vi "Buffer.vi"(7 "Cluster":T1={"JSON Buffer"="authtoken=239cf72879e39d0ce6e668cd5c3988b6&scope=creatorapi&zc_ownername=shanthapriya&XMLString=", "Server information start tag"="<ZohoCreator> <applicationlist> <application name='customer-application'><formlist>  <form name='EventLog'>", "Record start/end"="add", "Key name"="field name", "Value name"="value", "Server information end tag"="\"</form></formlist></application></applicationlist></ZohoCreator>"}, 8 "error in":errorcluster, 10 "Values":string[][](array[string]), 11 "Keys":string[](array[string])) -> (0 "Error out":errorcluster, 3 "Buffer":string)   [LabVIEW 2019, in "DataLogger.lvclass"]
doc: "Buffer"
uses:
  DataLogger.lvclass
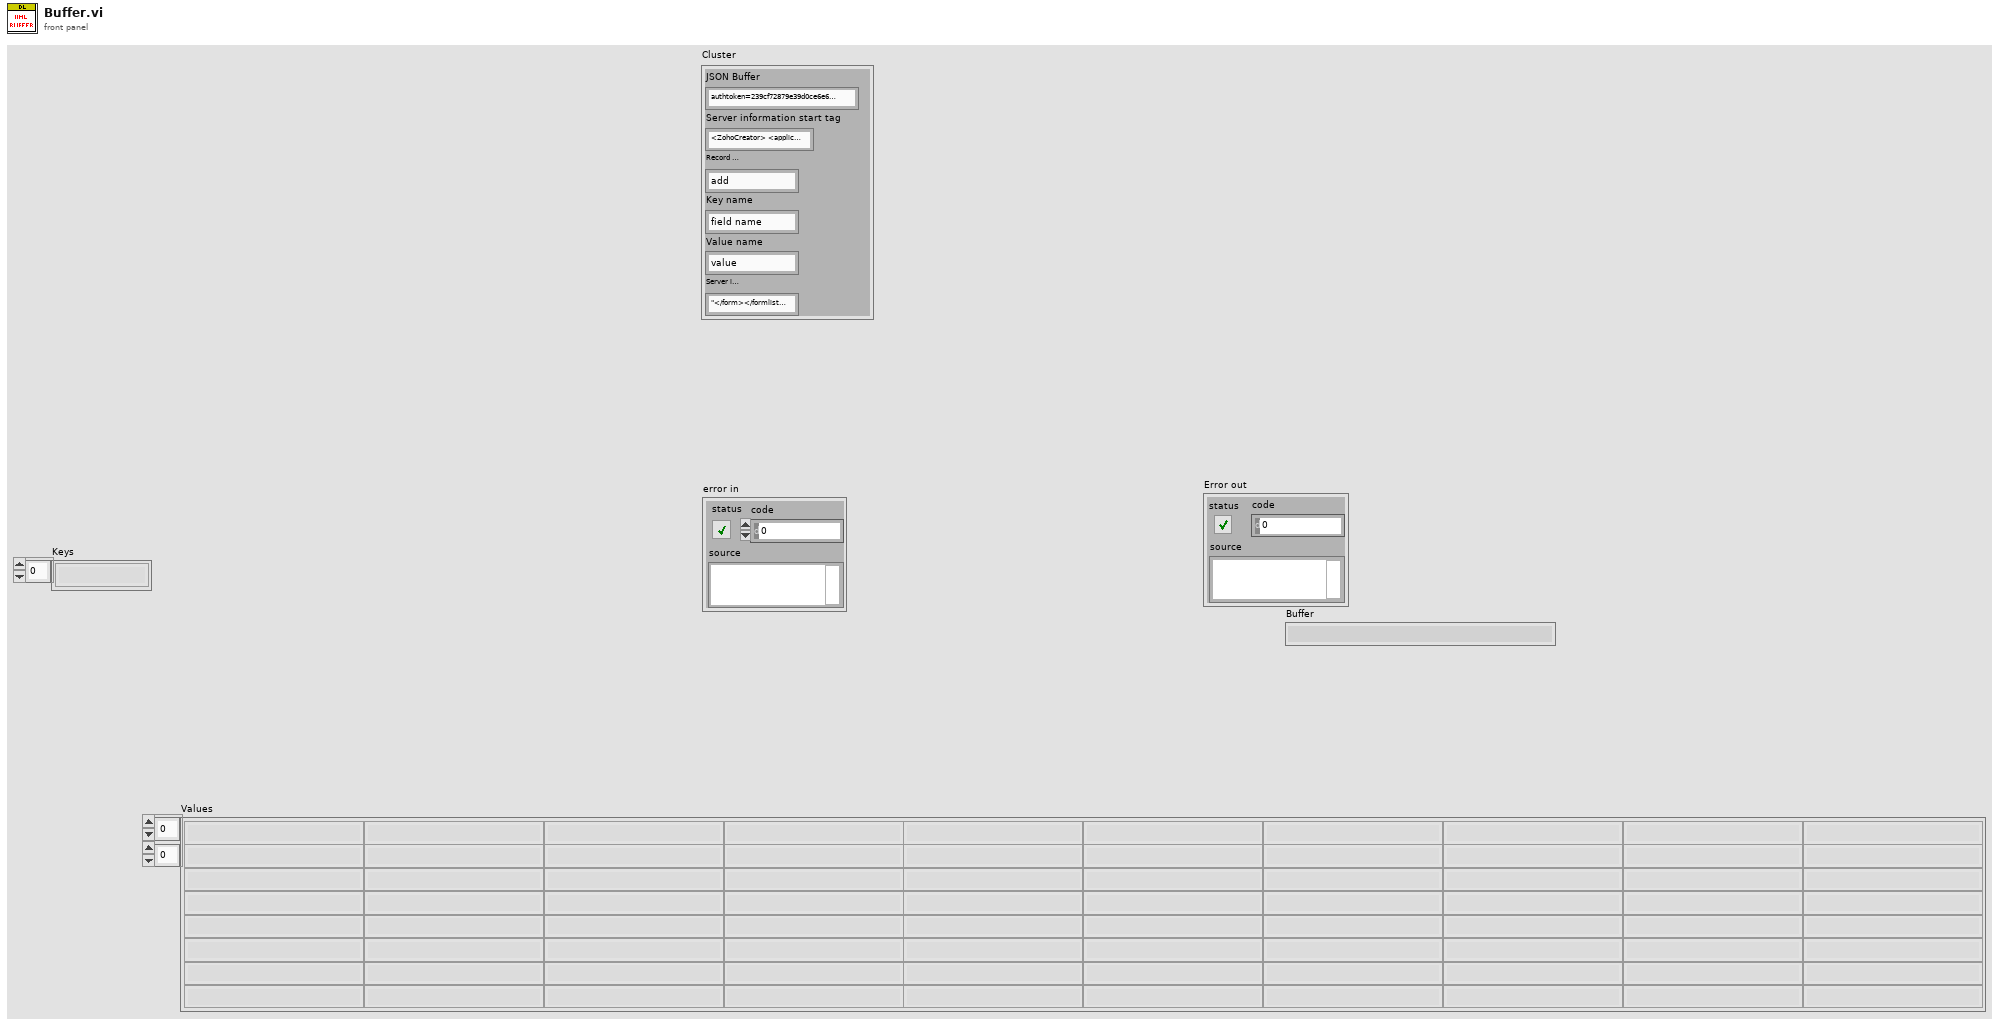
[diagram p1: front panel]
types:
  T1 = cluster{"JSON Buffer":string, "Server information start tag":string, "Record start/end":string, "Key name":string, "Value name":string, "Server information end tag":string}
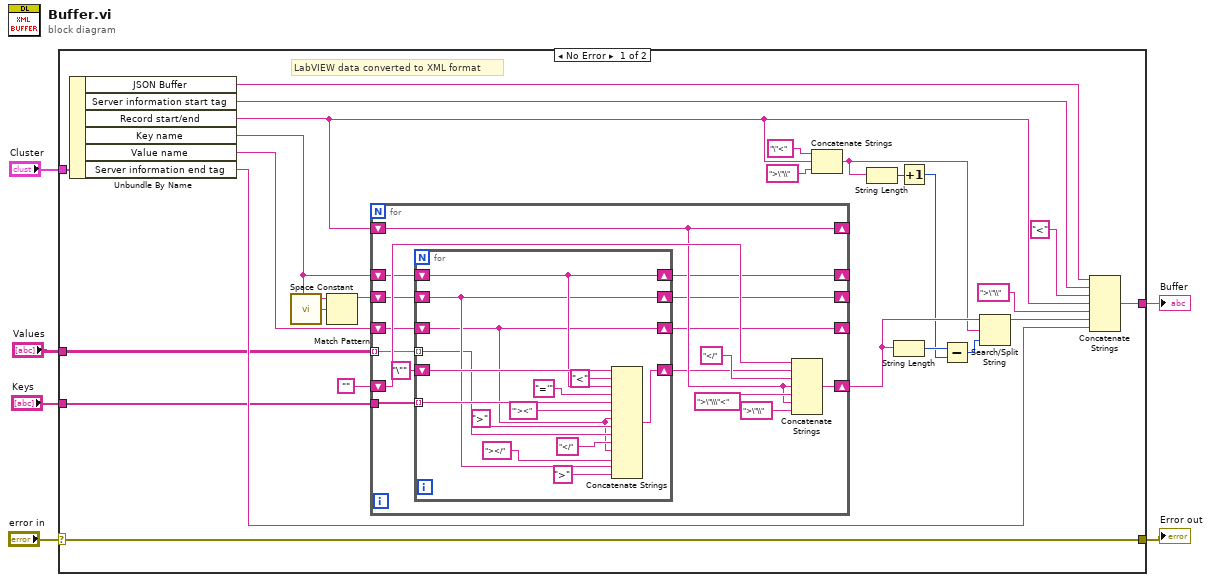
[diagram p0: block diagram]
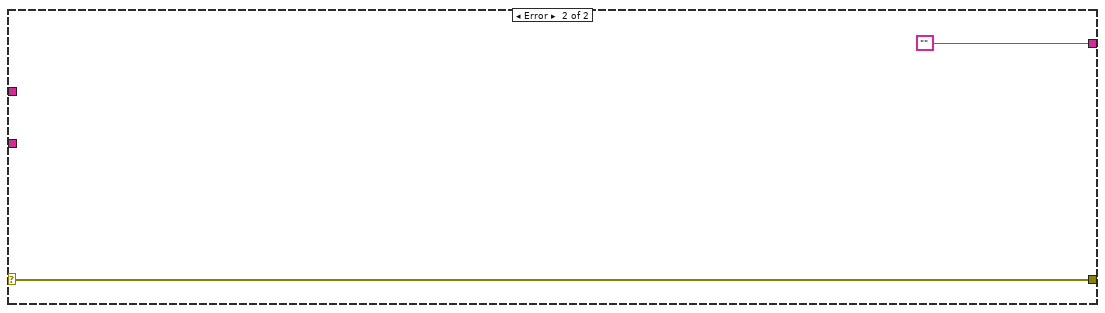
[diagram p2: hidden frame]
diagram:
  n1 = case shown="No Error" "error in" {
    selector: "error in" -> [w12 w63]
    tunnel: [w12 w63] -> w5
    tunnel: "Cluster" -> [w11 _]
    tunnel: "Keys" -> [w10 _]
    tunnel: "Values" -> [w9 _]
    tunnel: [w8 ""] -> w1
    frame No Error {
      # "LabVIEW data converted to XML format"
      n2 = Unbundle By Name(w11) -> ("JSON Buffer"=w27:string, "Server information start tag"=w28:string, "Record start/end"=w7:string, "Key name"=w13:string, "Value name"=w26:string, "Server information end tag"=w14:string)
      n3 = call <vilib>:"Space Constant.vi"() -> ("String"=w25:string)
      n4 = Match Pattern(string=w13, regular expression=w25) -> (before substring=w24:string)  [unwired: 1 in, 3 out]
      n5 = for {
        tunnel: w9 -> [w34] mode=indexing
        tunnel: w10 -> [w47]
        shift-right: [w45] -> w30
        shift-left: "" -> [w44]
        shift-right: [w38] -> _
        shift-left: w7 -> [w38]
        shift-right: [w36] -> _
        shift-left: w24 -> [w41]
        shift-right: [w32] -> _
        shift-left: w13 -> [w43]
        shift-right: [w35] -> _
        shift-left: w26 -> [w42]
        n6 = for {
          tunnel: w47 -> [w57] mode=indexing
          shift-right: [w50] -> w33
          shift-left: "\"" -> [w61]
          shift-right: [w59] -> w32
          shift-left: w43 -> [w59]
          shift-right: [w48] -> w35
          shift-left: w42 -> [w48]
          shift-right: [w52] -> w36
          shift-left: w41 -> [w52]
          tunnel: w34 -> [w49] mode=indexing
          n7 = Concatenate Strings(w61, "<" ("string"), w59, "='" ("string"), w57, "'><" ("string"), w48, ">" ("string"), w49, "</" ("string"), w48, "></" ("string"), w52, ">" ("string")) -> (w50:string)
        }
        n8 = Concatenate Strings(w44, w33, "</" ("string"), w38, ">\"\\\"<" ("string"), w38, ">\"\\" ("string")) -> (w45:string)
      }
      n9 = Concatenate Strings("\"<" ("string"), w7, ">\"\\" ("string")) -> (w20:string)
      n10 = String Length(string=w20) -> (length=w19:i32)
      n11 = String Length(string=w30) -> (length=w21:i32)
      n12 = Increment(x=w19) -> (x+1=w18:i32)
      n13 = Subtract(x=w21, y=w18) -> (x-y=w17:i32)
      n14 = Search/Split String(string=w30, search string/char (-)=w20, offset (0)=w17) -> (substring before match=w15:string)  [unwired: 2 out]
      n15 = Concatenate Strings(w27, w28, "<" ("string"), w7, ">\"\\" ("string"), w15, w14) -> (w8:string)
    }
    frame Error {
    }
  }
  "Error out" <- w5
  "Buffer" <- w1
